vi "Watlow.vi"() -> ()   [LabVIEW 2017]
uses:
  dll/Watbus.dll
  Type Def/Data.ctl
panel:
  out "Cool bench":dbl caption="Cool" format="%#_5g"
  out "Heat bench":dbl caption="Heat" format="%#_5g"
  out "Cool tripleur":dbl caption="Cool" format="%#_5g"
  out "Heat tripleur":dbl caption="Heat" format="%#_5g"
  out "Cool doubleur":dbl caption="Cool" format="%#_5g"
  out "Heat doubleur":dbl caption="Heat" format="%#_5g"
  out "COM port":i64
  out "error?":bool caption="erreur ?"
  out "User file contents Watlow":dbl[](array[numeric])
  out "file path":path
  out "valeur de l'horloge en ms":u32
  in  "Bouton Accueil":bool
  out "sortie d'erreur":errorcluster
  out "IsConnected":bool
  out "ILabVIEW":refnum<k24>
  out "error out 2":errorcluster
  out "Chaîne":string
  out "error IO":errorcluster
  out "Communications Port":refnum<visa-resource-name>
  in  "Start":bool
  out "Watlow file (1sec)":refnum<file>
  out "Tableau":dbl[][](array[numeric])
  out "Bench":dbl format="%#_5g"
  out "THG":dbl format="%#_5g"
  out "SHG":dbl format="%#_5g"
  in  "Stop":bool
  out "error out":errorcluster caption="sortie d'erreur"
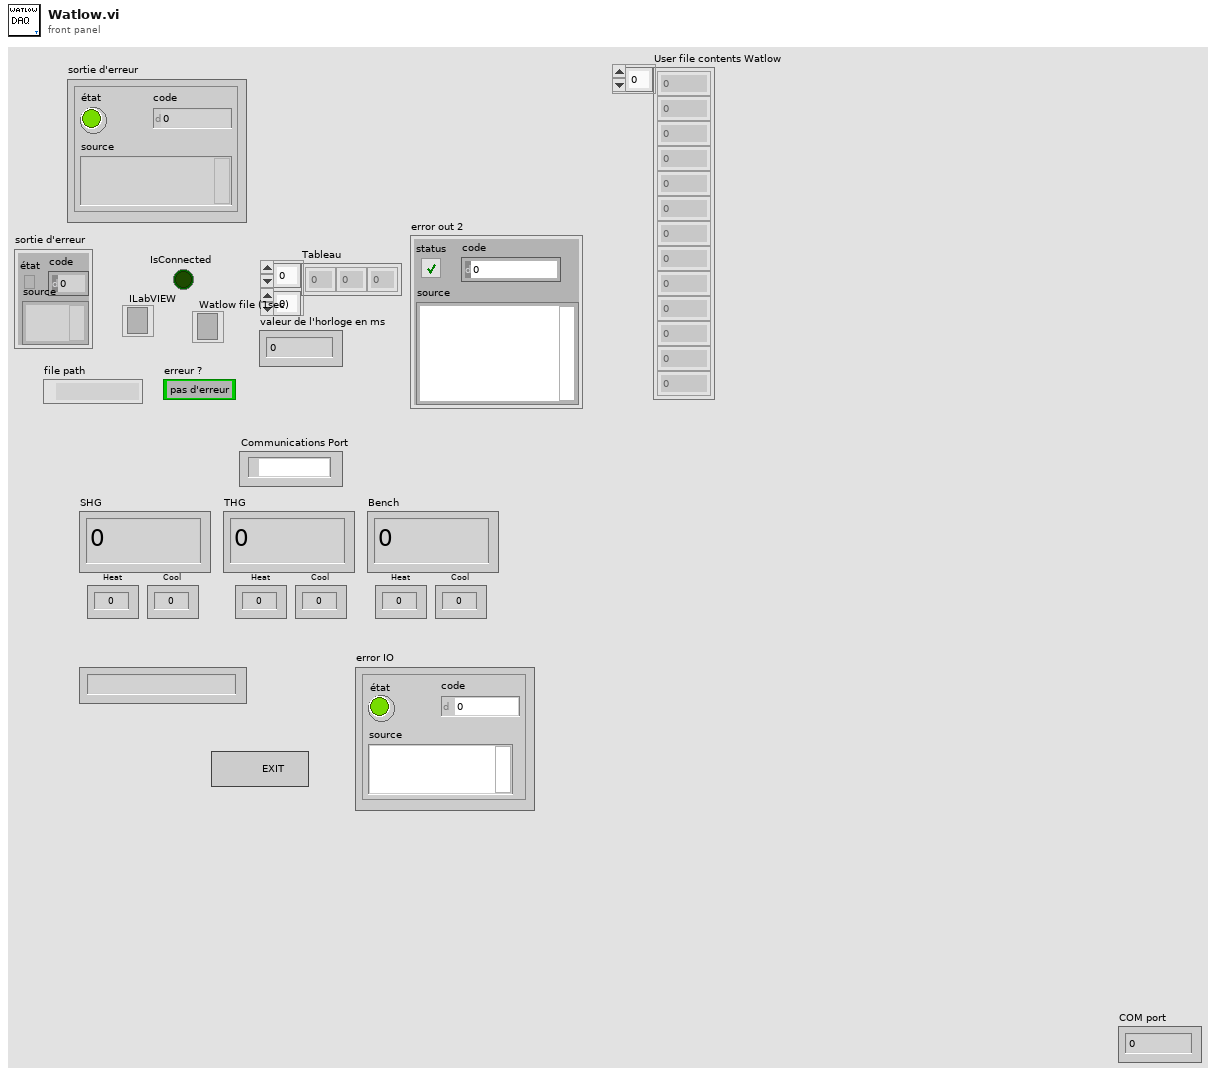
[diagram p1: front panel]
types:
  T1 = enum8{"Enabled", "Disabled", "Disabled and Grayed Out"}
  T2 = typedef "Data.ctl" = cluster{"Enum":enum16{"Init", "Read", "Stop"}, "Tableau":dbl[], "Date":string, "Time":u32}
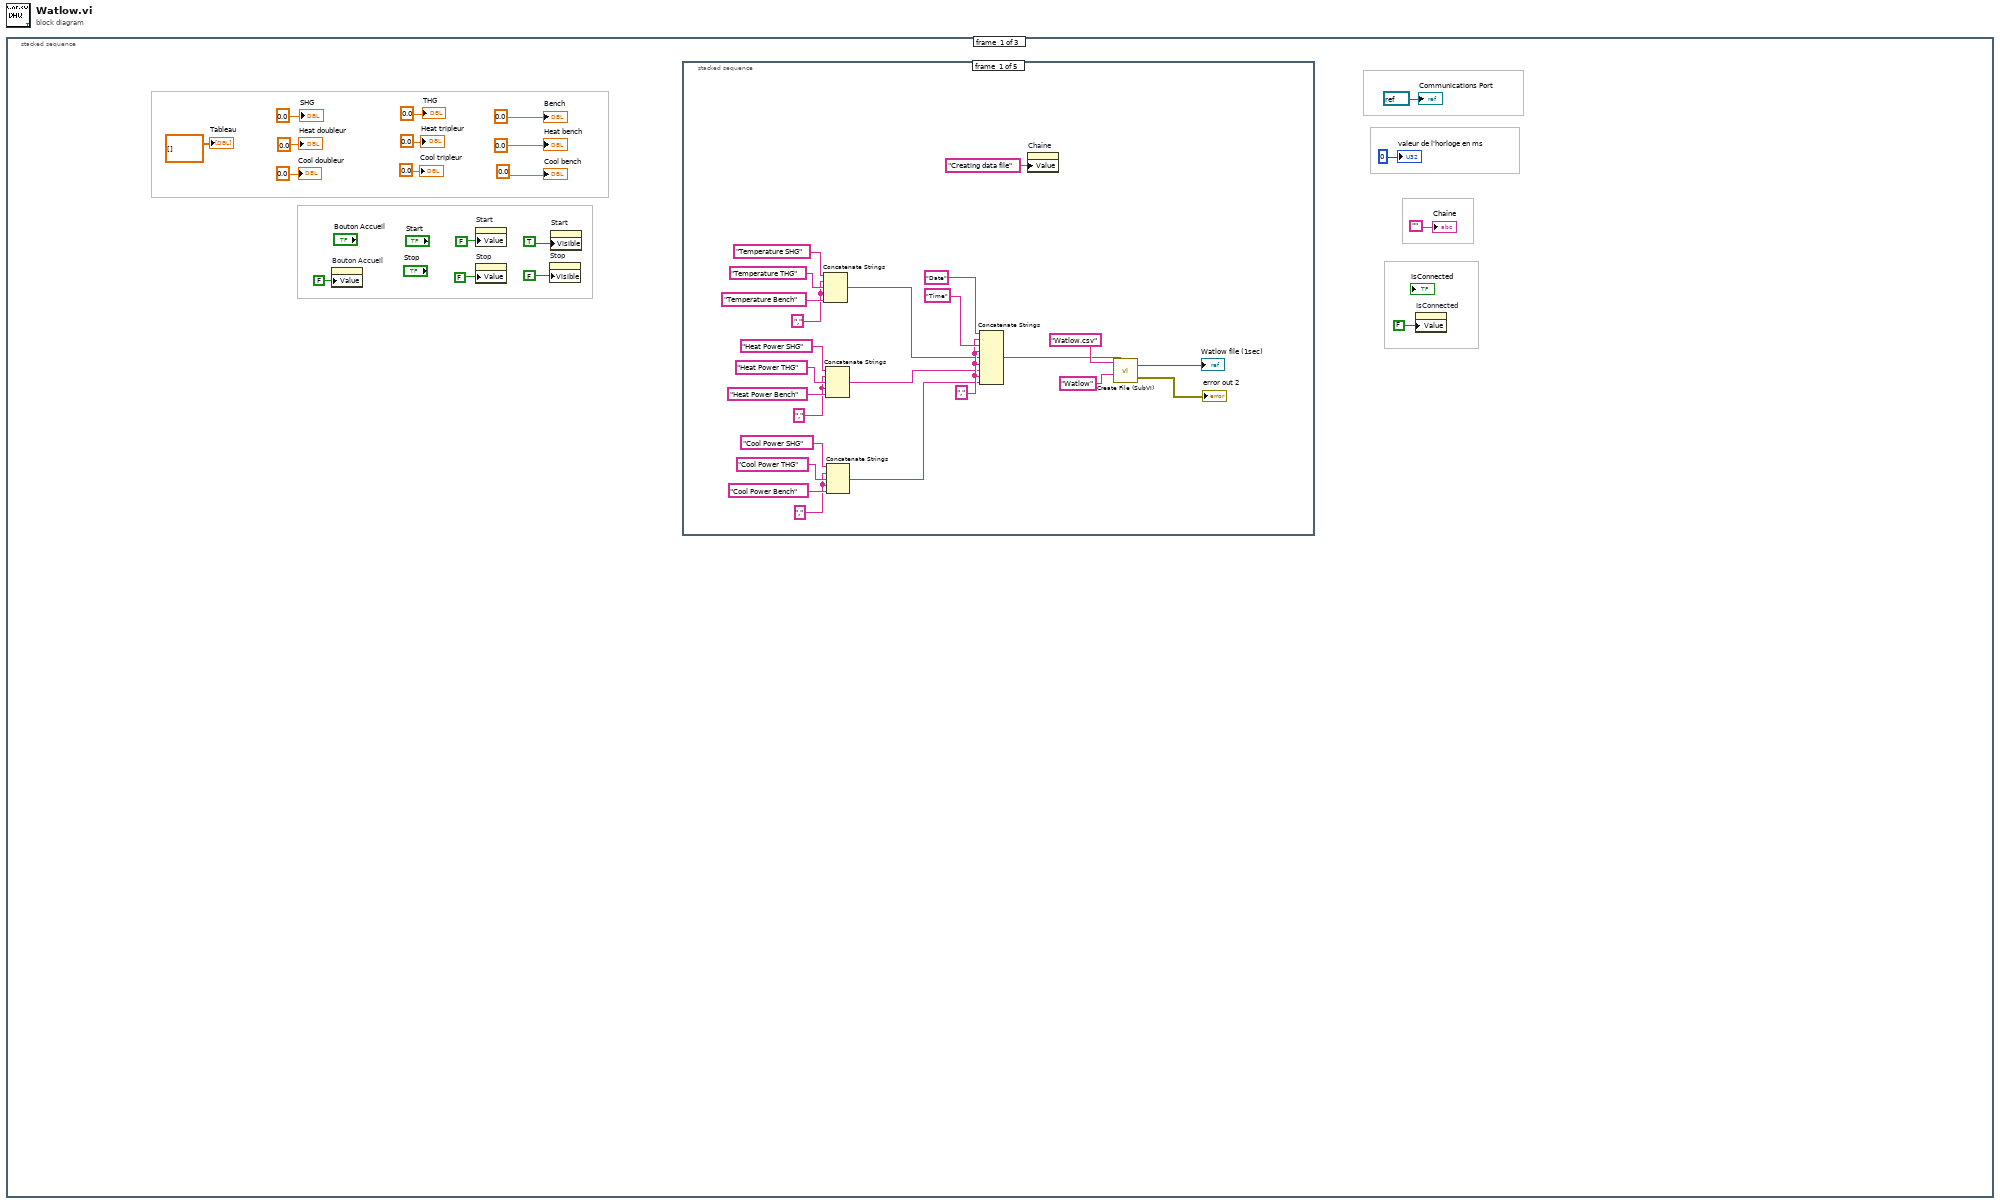
[diagram p0: block diagram]
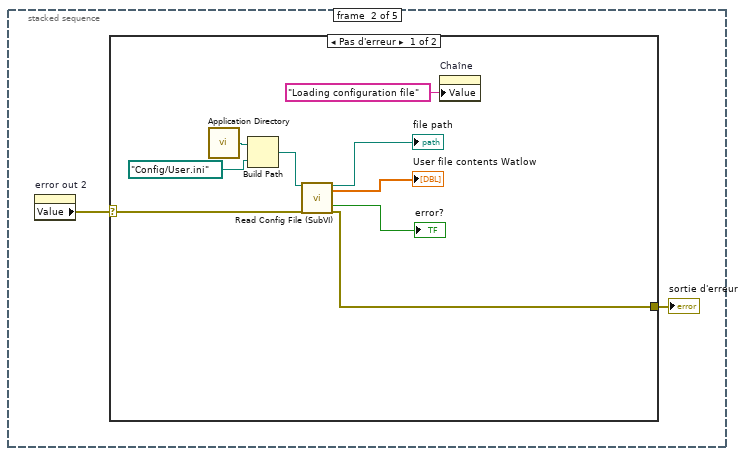
[diagram p2: hidden frame]
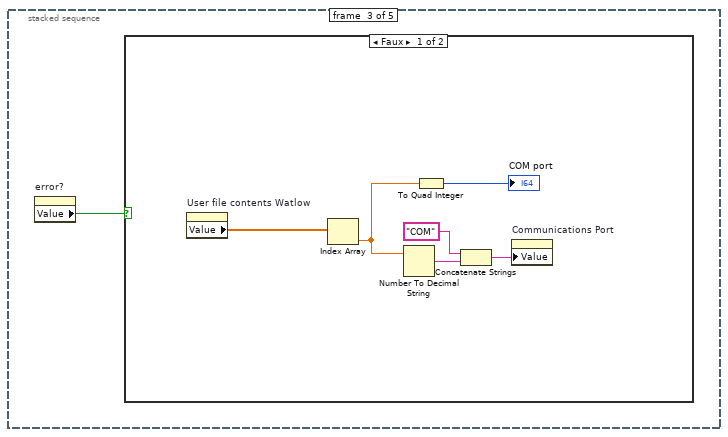
[diagram p4: hidden frame]
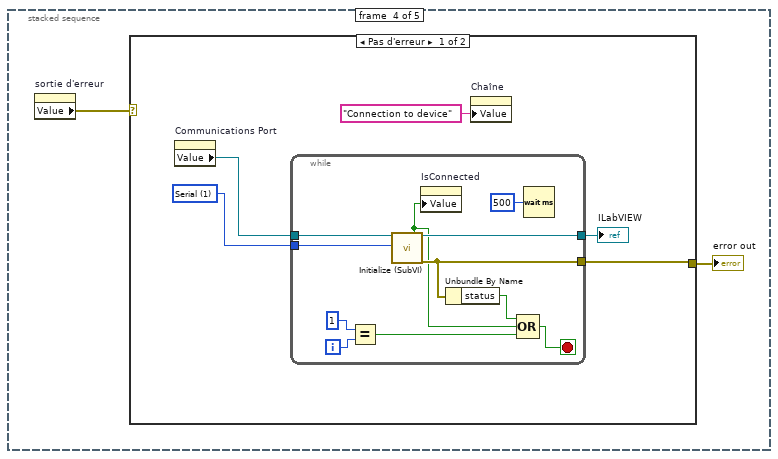
[diagram p6: hidden frame]
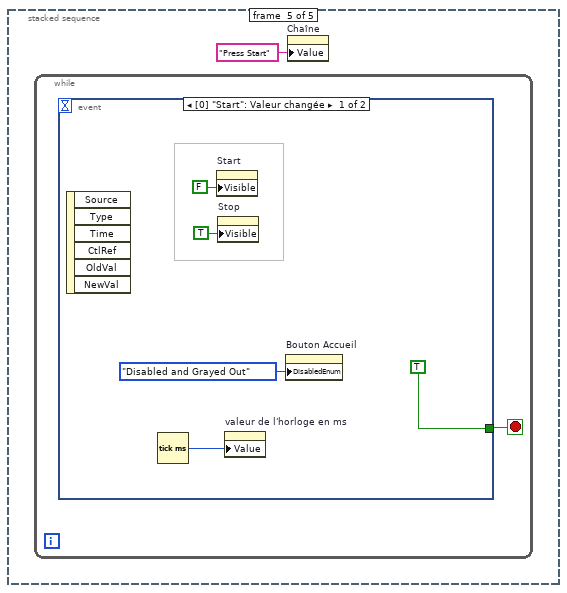
[diagram p8: hidden frame]
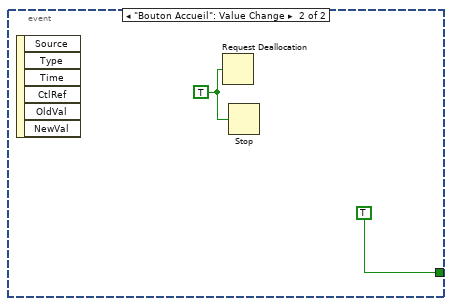
[diagram p9: hidden frame]
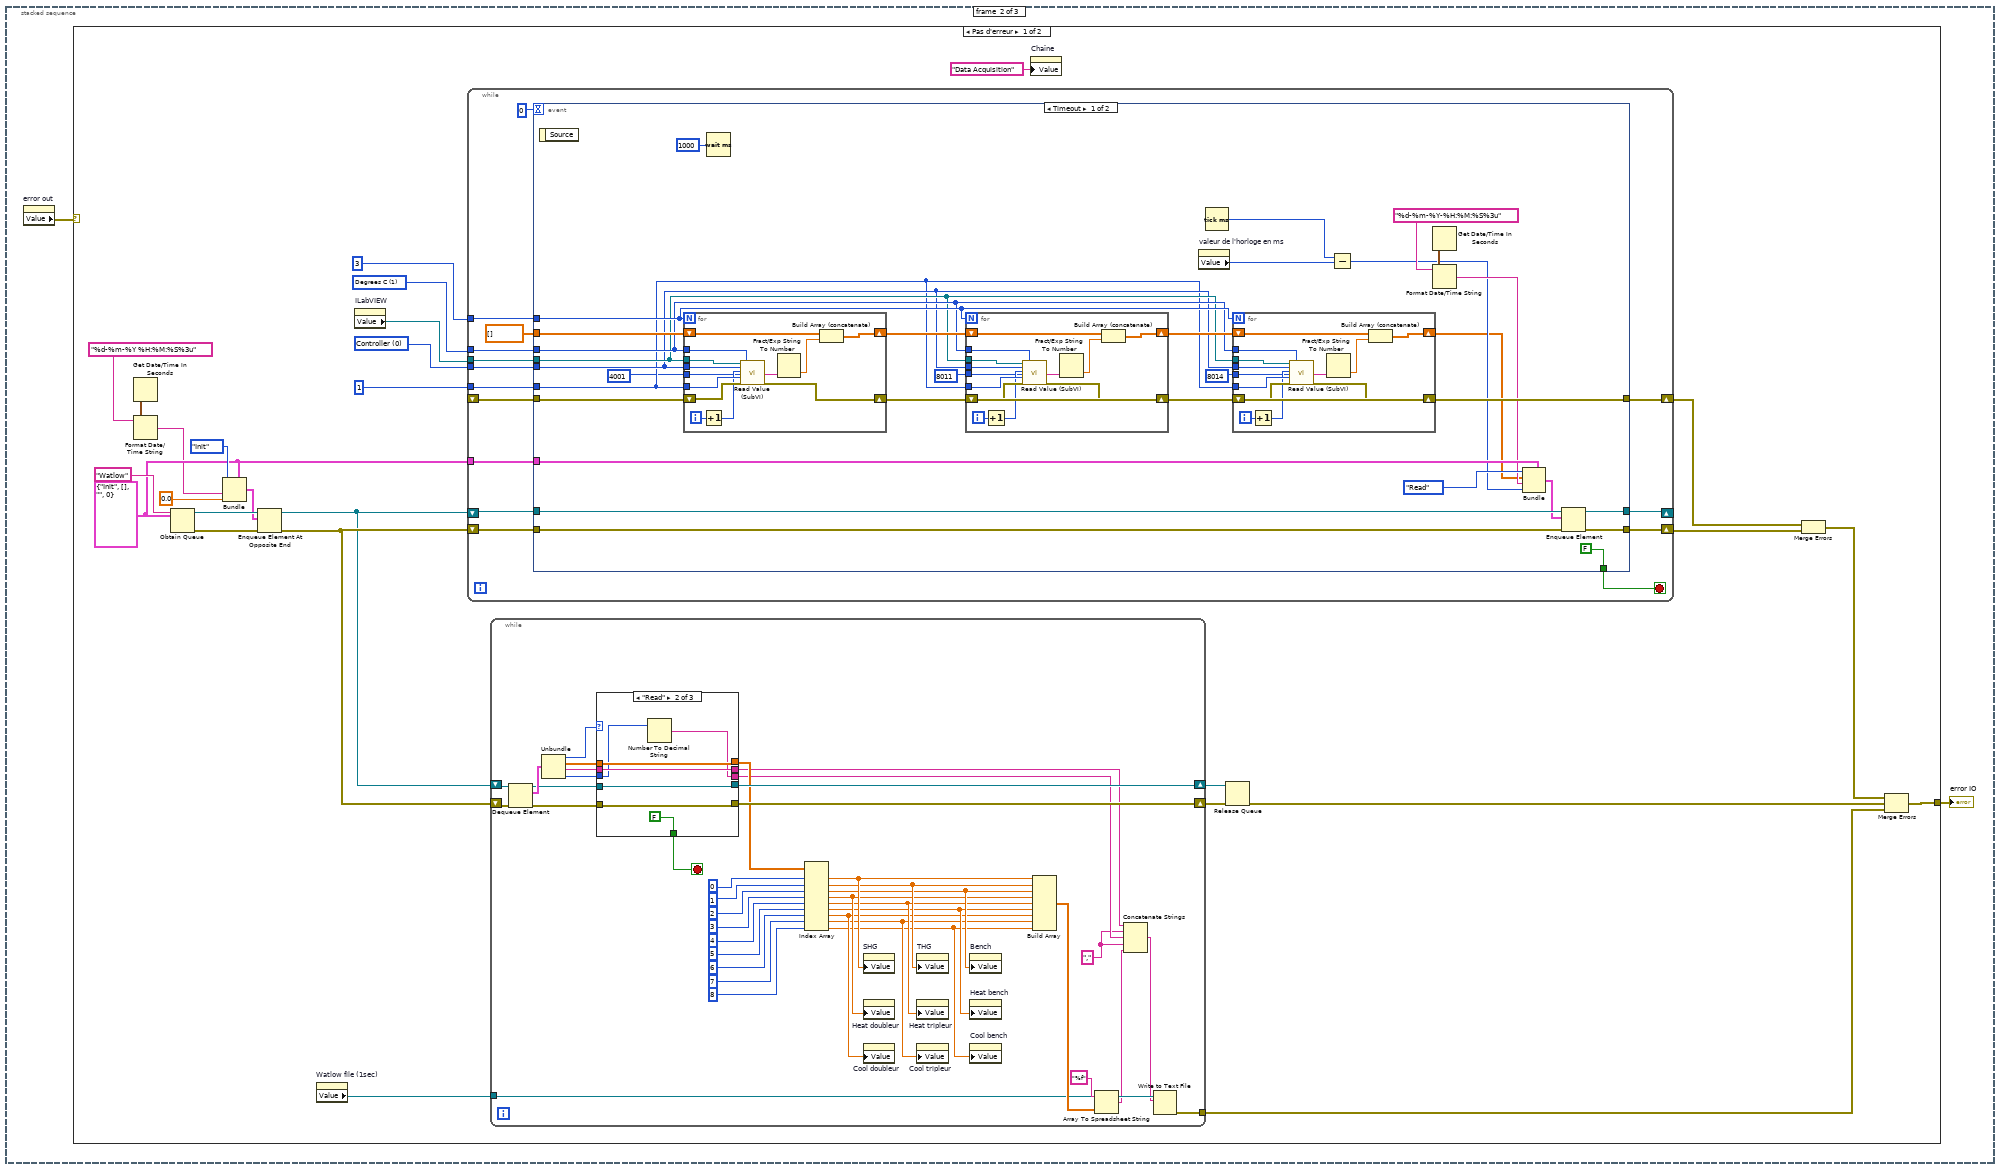
[diagram p10: hidden frame]
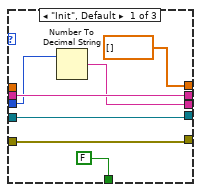
[diagram p11: hidden frame]
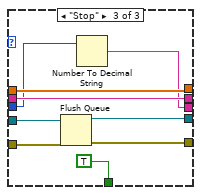
[diagram p12: hidden frame]
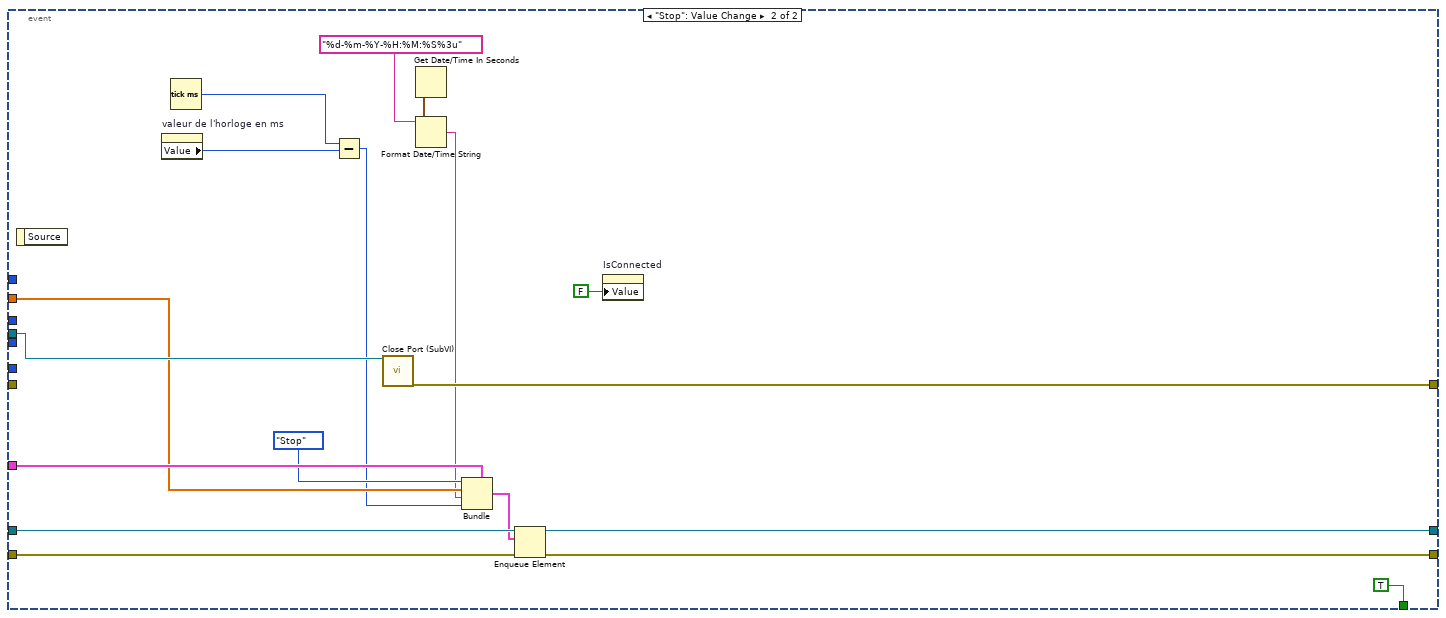
[diagram p13: hidden frame]
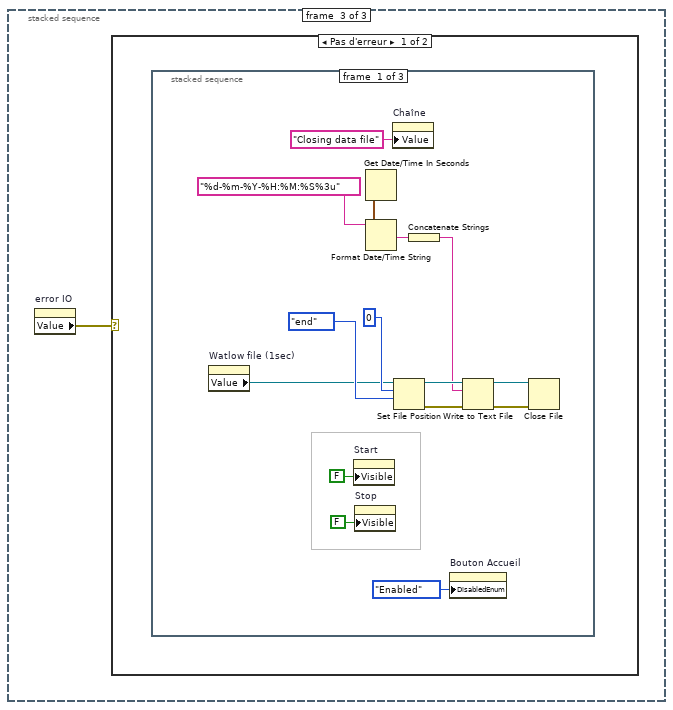
[diagram p15: hidden frame]
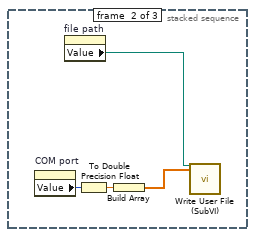
[diagram p16: hidden frame]
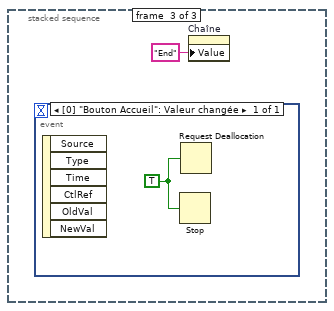
[diagram p17: hidden frame]
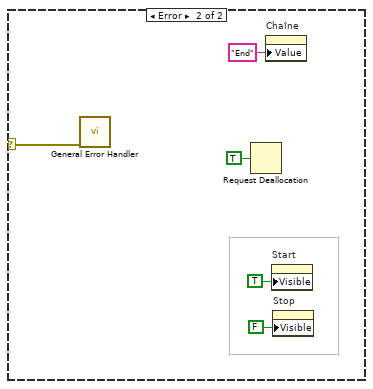
[diagram p18: hidden frame]
diagram:
  n1 = stacked-sequence {
    frame #0 {
      n2 = property on="Bouton Accueil" class="Bool (strict)"("Value"=FALSE ("Bouton Accueil")) -> ()  [unwired: 2 in, 2 out]
      n3 = property on="Start" class="Bool (strict)"("Value"=FALSE ("Start")) -> ()  [unwired: 2 in, 2 out]
      n4 = property on="Stop" class="Bool (strict)"("Value"=FALSE ("Bouton Stop")) -> ()  [unwired: 2 in, 2 out]
      n5 = property on="Stop" class="Bool (strict)"("Visible"=FALSE) -> ()  [unwired: 2 in, 2 out]
      n6 = property on="Start" class="Bool (strict)"("Visible"=TRUE) -> ()  [unwired: 2 in, 2 out]
      n7 = stacked-sequence {
        frame #0 {
          w22 = ","
          w26 = ","
          w31 = ","
          w36 = ","
          n8 = Concatenate Strings("Temperature SHG" ("chaîne"), w31, "Temperature THG" ("chaîne"), w31, "Temperature Bench" ("chaîne")) -> (w30:string)
          n9 = Concatenate Strings("Heat Power SHG" ("chaîne"), w26, "Heat Power THG" ("chaîne"), w26, "Heat Power Bench" ("chaîne")) -> (w21:string)
          n10 = Concatenate Strings("Cool Power SHG" ("chaîne"), w22, "Cool Power THG" ("chaîne"), w22, "Cool Power Bench" ("chaîne")) -> (w20:string)
          n11 = Concatenate Strings("Date" ("chaîne"), w36, "Time" ("chaîne"), w36, w30, w36, w21, w36, w20) -> (w38:string)
          n12 = property on="Chaîne" class="Ch"("Value"="Creating data file" ("Chaîne")) -> ()  [unwired: 2 in, 2 out]
          n13 = call "Create File (SubVI).vi"("headers"="Watlow" ("data name"), "data name"=w38, "file name"="Watlow.csv") -> ("error out"=→"error out 2":errorcluster, "Byte Stream File out"=→"Watlow file (1sec)":refnum<file>)  [unwired: 1 in]
        }
        frame #1 {
          n14 = property on="error out 2" class="Clust (strict)"() -> ("Value"=w45:errorcluster)  [unwired: 2 in, 2 out]
          n15 = case shown="Pas d'erreur" w45 {
            selector: w45 -> [w53 w55]
            tunnel: [w47 w55] -> w44
            frame No Error {
              n16 = call <vilib>:"Application Directory.vi"() -> ("Application Directory"=w52:path)
              n17 = Build Path(base path=w52, name or relative path=path "Config/User.ini") -> (appended path=w50:path)
              n18 = call "Read Config File (SubVI).vi"("configuration file path"=w50, "entrée d'erreur (pas d'erreur)"=w53) -> ("file path"=→"file path":path, "User file contents Watlow"=→"User file contents Watlow":dbl[], "error?"=→"error?":bool, "sortie d'erreur"=w47:errorcluster)  [unwired: 14 in]
              n19 = property on="Chaîne" class="Ch"("Value"="Loading configuration file" ("Chaîne")) -> ()  [unwired: 2 in, 2 out]
            }
            frame Error {
            }
          }
          "sortie d'erreur" <- w44
        }
        frame #2 {
          n20 = property on="error?" class="Bool (strict)"() -> ("Value"=w56:bool)  [unwired: 2 in, 2 out]
          n21 = case shown="Faux" w56 {
            frame False {
              n22 = property on="User file contents Watlow" class="Tabl (strict)"() -> ("Value"=w62:dbl[])  [unwired: 2 in, 2 out]
              n23 = Index Array(array=w62) -> (element=w58:dbl)  [unwired: 1 in]
              n24 = Number To Decimal String(number=w58) -> (decimal integer string=w60:string)  [unwired: 1 in]
              n25 = To Quad Integer(1:w58) -> (0:→"COM port":i64)
              n26 = Concatenate Strings("COM" ("string"), w60) -> (w57:string)
              n27 = property on="Communications Port" class="NomVISA"("Value"=w57) -> ()  [unwired: 2 in, 2 out]
            }
            frame True {
            }
          }
        }
        frame #3 {
          n28 = property on="sortie d'erreur" class="Clust (strict)"() -> ("Value"=w63:errorcluster)  [unwired: 2 in, 2 out]
          n29 = case shown="Pas d'erreur" w63 {
            selector: w63 -> [_ w81]
            tunnel: [w67 w81] -> w64
            frame No Error {
              w69 = 1 items=["Usb", "Serial", "Ethernet", "Unconnected"] ("InterfaceType")
              n30 = property on="Communications Port" class="NomVISA"() -> ("Value"=w65:refnum<visa-resource-name>)  [unwired: 2 in, 2 out]
              n31 = while {
                tunnel: [w73] -> w67
                tunnel: w69 -> [w80]
                tunnel: w65 -> [w71]
                tunnel: [w74] -> w66
                i -> [w78]
                stop <- w79 stop-if-true
                n32 = Equal?(x=1, y=w78) -> (x = y?=w76:bool)
                n33 = call "Initialize (SubVI).vi"("Communications Port"=w71, "InterfaceType"=w80) -> ("IsConnected"=w70:bool, "ILabVIEW"=w74:refnum<k24>, "error out"=w73:errorcluster)  [unwired: 15 in]
                n34 = property on="IsConnected" class="Bool (strict)"("Value"=w70) -> ()  [unwired: 2 in, 2 out]
                n35 = Unbundle By Name(w73) -> ("status"=w72:bool)
                n36 = Compound Arithmetic op=OR ("Opérateur arithmétique")(w72, w70, w76) -> (w79:bool)
                n37 = Wait (ms)(milliseconds to wait=u32 500 ("attente (ms)")) -> ()  [unwired: 1 out]
              }
              "ILabVIEW" <- w66
              n38 = property on="Chaîne" class="Ch"("Value"="Connection to device" ("Chaîne")) -> ()  [unwired: 2 in, 2 out]
            }
            frame Error {
            }
          }
          "error out" <- w64
        }
        frame #4 {
          n39 = while {
            stop <- w83 stop-if-true
            n40 = event shown="[0] \"Start\": Valeur changée" {
              selector: _ -> [_ _]
              dyn-events: _ -> [_ _]
              timeout: _ -> [_ _]
              tunnel: [TRUE TRUE] -> w83
              event "Start": Value Change {
                n41 = event-data() -> ()  [unwired: 1 in, 6 out]
                n42 = Tick Count (ms)() -> (millisecond timer value=w84:u32)
                n43 = property on="Start" class="Bool (strict)"("Visible"=FALSE) -> ()  [unwired: 2 in, 2 out]
                n44 = property on="Stop" class="Bool (strict)"("Visible"=TRUE) -> ()  [unwired: 2 in, 2 out]
                n45 = property on="valeur de l'horloge en ms" class="NumNb (strict)"("Value"=w84) -> ()  [unwired: 2 in, 2 out]
                n46 = property on="Bouton Accueil" class="Bool (strict)"("DisabledEnum"=T1."Disabled and Grayed Out" ("Désactivé")) -> ()  [unwired: 2 in, 2 out]
              }
              event "Bouton Accueil": Value Change {
                w90 = TRUE ("flag")
                n47 = event-data() -> ()  [unwired: 1 in, 6 out]
                n48 = Request Deallocation(w90) -> ()
                n49 = Stop(stop? (T)=w90) -> ()
              }
            }
          }
          n50 = property on="Chaîne" class="Ch"("Value"="Press Start" ("Chaîne")) -> ()  [unwired: 2 in, 2 out]
        }
      }
      n51 = property on="IsConnected" class="Bool (strict)"("Value"=FALSE ("IsConnected")) -> ()  [unwired: 2 in, 2 out]
      "SHG" <- 0.0 ("élément")
      "THG" <- 0.0 ("élément 2")
      "Bench" <- 0.0 ("élément 3")
      "Tableau" <- dbl[][] [] ("Tableau")
      "Chaîne" <- ""
      "Communications Port" <- refnum<visa-resource-name> refnum ("Communications Port")
      "valeur de l'horloge en ms" <- u32 0 ("valeur de l'horloge en ms")
      "Heat doubleur" <- 0.0 ("Heat doubleur")
      "Cool doubleur" <- 0.0 ("Cool doubleur")
      "Heat tripleur" <- 0.0 ("Heat tripleur")
      "Cool tripleur" <- 0.0 ("Cool tripleur")
      "Heat bench" <- 0.0 ("Heat bench")
      "Cool bench" <- 0.0 ("Cool bench")
    }
    frame #1 {
      n52 = property on="error out" class="Clust (strict)"() -> ("Value"=w92:errorcluster)  [unwired: 2 in, 2 out]
      n53 = case shown="Pas d'erreur" w92 {
        selector: w92 -> [_ w284]
        tunnel: [w106 w284] -> w91
        frame No Error {
          w117 = 0 items=["Controller", "RUI", "PC", "CommsCard"] ("DeviceType")
          w118 = u8 1 items=["Degrees F", "Degrees C"] ("TemperatureUnits")
          w97 = T2 {"Enum"=enum."Init", "Tableau"=[], "Date"="", "Time"=0} ("Enum")
          n54 = Get Date/Time In Seconds() -> (seconds since 1Jan1904=w96:timestamp)
          n55 = Format Date/Time String(time format string (%c)="%d-%m-%Y %H:%M:%S%3u", seconds (now)=w96) -> (date/time string=w94:string)  [unwired: 1 in]
          n56 = Obtain Queue(name (unnamed)="Watlow" ("nom (aucun)"), element data type=w97) -> (queue out=w100:refnum<queue>, error out=w103:errorcluster)  [unwired: 3 in, 1 out]
          n57 = Bundle(cluster=w97, "Enum"=enum16{"Init", "Read", "Stop"}."Init", "Date"=w94, "Time"=0.0) -> (w98:T2)  [unwired: 1 in]
          n58 = Enqueue Element At Opposite End(queue=w100, element=w98, error in (no error)=w103) -> (queue out=w101:refnum<queue>, error out=w102:errorcluster)  [unwired: 1 in, 1 out]
          n59 = property on="Watlow file (1sec)" class="Ref (strict)"() -> ("Value"=w107:refnum<file>)  [unwired: 2 in, 2 out]
          n60 = property on="ILabVIEW" class="Ref (strict)"() -> ("Value"=w104:refnum<k24>)  [unwired: 2 in, 2 out]
          n61 = while {
            shift-right: [w196] -> w111
            shift-left: w102 -> [w197]
            shift-right: [w194] -> _
            shift-left: w101 -> [w195]
            tunnel: w118 -> [w193]
            tunnel: w117 -> [w192]
            tunnel: 1 ("InstanceId") -> [w191]
            tunnel: 3 -> [w190]
            shift-right: [w188] -> w112
            shift-left: _ -> [w189]
            tunnel: w97 -> [w187]
            tunnel: w104 -> [w184]
            stop <- w186 stop-if-true
            n62 = event shown="[0] Timeout" {
              selector: _ -> [_ _]
              dyn-events: _ -> [_ _]
              timeout: 0 -> [_ _]
              tunnel: w197 -> [w224 w281]
              tunnel: [w223 w280] -> w196
              tunnel: w195 -> [w226 w282]
              tunnel: [w225 w279] -> w194
              tunnel: w193 -> [w204 _]
              tunnel: w192 -> [w202 _]
              tunnel: w191 -> [w201 _]
              tunnel: w190 -> [w208 _]
              tunnel: w189 -> [w222 _]
              tunnel: [w221 w275] -> w188
              tunnel: w187 -> [w220 w277]
              tunnel: [FALSE TRUE] -> w186
              tunnel: w184 -> [w203 w274]
              tunnel: dbl[] [] -> [w216 w272]
              event Timeout {
                n63 = event-data() -> ()  [unwired: 1 in, 1 out]
                n64 = for {
                  N: w208 -> [_]
                  tunnel: w204 -> [w265]
                  tunnel: w202 -> [w264]
                  tunnel: w201 -> [w263]
                  shift-right: [w260] -> w221
                  shift-left: w222 -> [w261]
                  shift-right: [w256] -> w205
                  shift-left: w216 -> [w255]
                  tunnel: w203 -> [w254]
                  tunnel: 4001 ("ParameterID") -> [w253]
                  i -> [w262]
                  n65 = Increment(x=w262) -> (x+1=w258:i32)
                  n66 = call "Read Value (SubVI).vi"("ILabVIEW In"=w254, "DeviceType"=w264, "Zone"=w258, "ParameterID"=w253, "InstanceId"=w263, "error in (no error)"=w261, "TemperatureUnits"=w265) -> ("Value Out"=w259:string, "error out"=w260:errorcluster)  [unwired: 10 in, 1 out]
                  n67 = Fract/Exp String To Number(string=w259) -> (number=w257:dbl)  [unwired: 3 in, 1 out]
                  n68 = Build Array (concatenate)(w255, w257) -> (w256:dbl[])
                }
                n69 = Wait (ms)(milliseconds to wait=u32 1000 ("attente (ms)")) -> ()  [unwired: 1 out]
                n70 = for {
                  N: w208 -> [_]
                  tunnel: w204 -> [w252]
                  tunnel: w202 -> [w251]
                  tunnel: w201 -> [w250]
                  shift-right: [w247] -> _
                  shift-left: _ -> [w248]
                  shift-right: [w243] -> w206
                  shift-left: w205 -> [w242]
                  tunnel: w203 -> [w241]
                  tunnel: 8011 -> [w240]
                  i -> [w249]
                  n71 = Increment(x=w249) -> (x+1=w245:i32)
                  n72 = call "Read Value (SubVI).vi"("ILabVIEW In"=w241, "DeviceType"=w251, "Zone"=w245, "ParameterID"=w240, "InstanceId"=w250, "error in (no error)"=w248, "TemperatureUnits"=w252) -> ("Value Out"=w246:string, "error out"=w247:errorcluster)  [unwired: 10 in, 1 out]
                  n73 = Fract/Exp String To Number(string=w246) -> (number=w244:dbl)  [unwired: 3 in, 1 out]
                  n74 = Build Array (concatenate)(w242, w244) -> (w243:dbl[])
                }
                n75 = property on="valeur de l'horloge en ms" class="NumNb (strict)"() -> ("Value"=w211:u32)  [unwired: 2 in, 2 out]
                n76 = Tick Count (ms)() -> (millisecond timer value=w212:u32)
                n77 = for {
                  N: w208 -> [_]
                  tunnel: w204 -> [w239]
                  tunnel: w202 -> [w238]
                  tunnel: w201 -> [w237]
                  shift-right: [w234] -> _
                  shift-left: _ -> [w235]
                  shift-right: [w230] -> w207
                  shift-left: w206 -> [w229]
                  tunnel: w203 -> [w228]
                  tunnel: 8014 -> [w227]
                  i -> [w236]
                  n78 = Increment(x=w236) -> (x+1=w232:i32)
                  n79 = call "Read Value (SubVI).vi"("ILabVIEW In"=w228, "DeviceType"=w238, "Zone"=w232, "ParameterID"=w227, "InstanceId"=w237, "error in (no error)"=w235, "TemperatureUnits"=w239) -> ("Value Out"=w233:string, "error out"=w234:errorcluster)  [unwired: 10 in, 1 out]
                  n80 = Fract/Exp String To Number(string=w233) -> (number=w231:dbl)  [unwired: 3 in, 1 out]
                  n81 = Build Array (concatenate)(w229, w231) -> (w230:dbl[])
                }
                n82 = Subtract(x=w212, y=w211) -> (x-y=w210:u32)
                n83 = Get Date/Time In Seconds() -> (seconds since 1Jan1904=w215:timestamp)
                n84 = Format Date/Time String(time format string (%c)="%d-%m-%Y-%H:%M:%S%3u", seconds (now)=w215) -> (date/time string=w213:string)  [unwired: 1 in]
                n85 = Bundle(cluster=w220, "Enum"=enum16{"Init", "Read", "Stop"}."Read", "Tableau"=w207, "Date"=w213, "Time"=w210) -> (w219:T2)
                n86 = Enqueue Element(queue=w226, element=w219, error in (no error)=w224) -> (queue out=w225:refnum<queue>, error out=w223:errorcluster)  [unwired: 1 in, 1 out]
              }
              event "Stop": Value Change {
                n87 = event-data() -> ()  [unwired: 1 in, 1 out]
                n88 = property on="valeur de l'horloge en ms" class="NumNb (strict)"() -> ("Value"=w267:u32)  [unwired: 2 in, 2 out]
                n89 = Tick Count (ms)() -> (millisecond timer value=w268:u32)
                n90 = Subtract(x=w268, y=w267) -> (x-y=w266:u32)
                n91 = call "Close Port (SubVI).vi"("ILabVIEW In"=w274) -> ("error out"=w275:errorcluster)  [unwired: 18 in]
                n92 = Get Date/Time In Seconds() -> (seconds since 1Jan1904=w271:timestamp)
                n93 = Format Date/Time String(time format string (%c)="%d-%m-%Y-%H:%M:%S%3u", seconds (now)=w271) -> (date/time string=w269:string)  [unwired: 1 in]
                n94 = Bundle(cluster=w277, "Enum"=enum16{"Init", "Read", "Stop"}."Stop", "Tableau"=w272, "Date"=w269, "Time"=w266) -> (w278:T2)
                n95 = Enqueue Element(queue=w282, element=w278, error in (no error)=w281) -> (queue out=w279:refnum<queue>, error out=w280:errorcluster)  [unwired: 1 in, 1 out]
                n96 = property on="IsConnected" class="Bool (strict)"("Value"=FALSE ("IsConnected")) -> ()  [unwired: 2 in, 2 out]
              }
            }
          }
          n97 = while {
            shift-right: [w151] -> w114
            shift-left: w101 -> [w158]
            shift-right: [w152] -> w113
            shift-left: w102 -> [w159]
            tunnel: [w143] -> w108
            tunnel: w107 -> [w142]
            stop <- w150 stop-if-true
            w135 = ","
            n98 = Dequeue Element(queue=w158, error in (no error)=w159) -> (queue out=w154:refnum<queue>, element=w157:T2, error out=w153:errorcluster)  [unwired: 1 in, 1 out]
            n99 = Unbundle(w157) -> ("Enum"=w156:enum16{"Init", "Read", "Stop"}, "Tableau"=w155:dbl[], "Date"=w140:string, "Time"=w139:u32)
            n100 = case shown="\"Read\"" w156 {
              tunnel: w155 -> [_ w170 w177]
              tunnel: w154 -> [w166 w173 w182]
              tunnel: w153 -> [w165 w172 w181]
              tunnel: [w165 w172 w180] -> w152
              tunnel: [w166 w173 w179] -> w151
              tunnel: [FALSE FALSE TRUE] -> w150
              tunnel: [dbl[] [] w170 w177] -> w146
              tunnel: [w162 w169 w176] -> w137
              tunnel: w140 -> [w162 w169 w176]
              tunnel: w139 -> [w161 w168 w175]
              tunnel: [w160 w167 w174] -> w138
              frame "Init", Default {
                n101 = Number To Decimal String(number=w161) -> (decimal integer string=w160:string)  [unwired: 1 in]
              }
              frame "Read" {
                n102 = Number To Decimal String(number=w168) -> (decimal integer string=w167:string)  [unwired: 1 in]
              }
              frame "Stop" {
                n103 = Flush Queue(queue=w182, error in (no error)=w181) -> (queue out=w179:refnum<queue>, error out=w180:errorcluster)  [unwired: 1 out]
                n104 = Number To Decimal String(number=w175) -> (decimal integer string=w174:string)  [unwired: 1 in]
              }
            }
            n105 = Index Array(array=w146, index #1=0 ("indice"), index #2=1 ("indice"), index #3=2 ("indice"), index #4=3 ("indice"), index #5=4 ("indice"), index #6=5 ("indice"), index #7=6 ("indice"), index #8=7 ("indice"), index #9=8 ("indice")) -> (element #1=w128:dbl, element #2=w127:dbl, element #3=w126:dbl, element #4=w125:dbl, element #5=w124:dbl, element #6=w123:dbl, element #7=w122:dbl, element #8=w121:dbl, element #9=w120:dbl)
            n106 = property on="SHG" class="NumNb (strict)"("Value"=w128) -> ()  [unwired: 2 in, 2 out]
            n107 = property on="Heat doubleur" class="NumNb (strict)"("Value"=w125) -> ()  [unwired: 2 in, 2 out]
            n108 = property on="Cool doubleur" class="NumNb (strict)"("Value"=w122) -> ()  [unwired: 2 in, 2 out]
            n109 = property on="THG" class="NumNb (strict)"("Value"=w127) -> ()  [unwired: 2 in, 2 out]
            n110 = property on="Heat tripleur" class="NumNb (strict)"("Value"=w124) -> ()  [unwired: 2 in, 2 out]
            n111 = property on="Cool tripleur" class="NumNb (strict)"("Value"=w121) -> ()  [unwired: 2 in, 2 out]
            n112 = property on="Bench" class="NumNb (strict)"("Value"=w126) -> ()  [unwired: 2 in, 2 out]
            n113 = property on="Heat bench" class="NumNb (strict)"("Value"=w123) -> ()  [unwired: 2 in, 2 out]
            n114 = property on="Cool bench" class="NumNb (strict)"("Value"=w120) -> ()  [unwired: 2 in, 2 out]
            n115 = Build Array(w128, w127, w126, w125, w124, w123, w122, w121, w120) -> (w144:dbl[])
            n116 = Array To Spreadsheet String(array=w144, 3:"%f" ("chaîne de format")) -> (spreadsheet string=w136:string)  [unwired: 1 in]
            n117 = Concatenate Strings(w137, w135, w138, w135, w136) -> (w141:string)
            n118 = Write to Text File(file (use dialog)=w142, text=w141) -> (error out=w143:errorcluster)  [unwired: 2 in, 2 out]
          }
          n119 = property on="Chaîne" class="Ch"("Value"="Data Acquisition" ("Chaîne")) -> ()  [unwired: 2 in, 2 out]
          n120 = Release Queue(queue=w114, error in (no error)=w113) -> (error out=w110:errorcluster)  [unwired: 1 in, 2 out]
          n121 = Merge Errors(w112, w111) -> (w109:errorcluster)
          n122 = Merge Errors(w109, w110, w108) -> (w106:errorcluster)
        }
        frame Error {
        }
      }
      "error IO" <- w91
    }
    frame #2 {
      n123 = property on="error IO" class="Clust (strict)"() -> ("Value"=w285:errorcluster)  [unwired: 2 in, 2 out]
      n124 = case shown="Pas d'erreur" w285 {
        selector: w285 -> [_ w309]
        frame No Error {
          n125 = stacked-sequence {
            frame #0 {
              n126 = property on="Watlow file (1sec)" class="Ref (strict)"() -> ("Value"=w292:refnum<file>)  [unwired: 2 in, 2 out]
              n127 = property on="Start" class="Bool (strict)"("Visible"=FALSE) -> ()  [unwired: 2 in, 2 out]
              n128 = property on="Stop" class="Bool (strict)"("Visible"=FALSE) -> ()  [unwired: 2 in, 2 out]
              n129 = Get Date/Time In Seconds() -> (seconds since 1Jan1904=w298:timestamp)
              n130 = Format Date/Time String(time format string (%c)="%d-%m-%Y-%H:%M:%S%3u", seconds (now)=w298) -> (date/time string=w296:string)  [unwired: 1 in]
              n131 = property on="Chaîne" class="Ch"("Value"="Closing data file" ("Chaîne")) -> ()  [unwired: 2 in, 2 out]
              n132 = Set File Position(offset (in bytes) (0)=i64 0 ("offset (en octets) (0)"), refnum=w292, from (0:start)=enum16{"start", "end", "current"}."end" ("à partir de (0 : start)")) -> (refnum out=w299:refnum<file>, error out=w288:errorcluster)  [unwired: 1 in]
              n133 = Concatenate Strings(w296) -> (w295:string)
              n134 = property on="Bouton Accueil" class="Bool (strict)"("DisabledEnum"=T1."Enabled" ("Désactivé")) -> ()  [unwired: 2 in, 2 out]
              n135 = Write to Text File(file (use dialog)=w299, text=w295, error in=w288) -> (refnum out=w300:refnum<file>, error out=w287:errorcluster)  [unwired: 1 in, 1 out]
              n136 = Close File(refnum=w300, error in=w287) -> ()  [unwired: 2 out]
            }
            frame #1 {
              n137 = property on="COM port" class="NumNb (strict)"() -> ("Value"=w304:i64)  [unwired: 2 in, 2 out]
              n138 = property on="file path" class="Chm"() -> ("Value"=w301:path)  [unwired: 2 in, 2 out]
              n139 = To Double Precision Float(number=w304) -> (double precision float=w302:dbl)
              n140 = Build Array(w302) -> (w303:dbl[])
              n141 = call "Write User File (SubVI).vi"("configuration file path"=w301, "User file contents Watlow"=w303) -> ()  [unwired: 24 in, 2 out]
            }
            frame #2 {
              n142 = event shown="[0] \"Bouton Accueil\": Valeur changée" {
                selector: _ -> [_]
                dyn-events: _ -> [_]
                timeout: _ -> [_]
                event "Bouton Accueil": Value Change {
                  w306 = TRUE ("flag")
                  n143 = event-data() -> ()  [unwired: 1 in, 6 out]
                  n144 = Stop(stop? (T)=w306) -> ()
                  n145 = Request Deallocation(w306) -> ()
                }
              }
              n146 = property on="Chaîne" class="Ch"("Value"="End" ("Chaîne")) -> ()  [unwired: 2 in, 2 out]
            }
          }
        }
        frame Error {
          n147 = call <vilib>:"General Error Handler.vi"("error in (no error)"=w309) -> ()  [unwired: 10 in, 5 out]
          n148 = Request Deallocation(TRUE ("flag")) -> ()
          n149 = property on="Chaîne" class="Ch"("Value"="End" ("Chaîne")) -> ()  [unwired: 2 in, 2 out]
          n150 = property on="Start" class="Bool (strict)"("Visible"=TRUE) -> ()  [unwired: 2 in, 2 out]
          n151 = property on="Stop" class="Bool (strict)"("Visible"=FALSE) -> ()  [unwired: 2 in, 2 out]
        }
      }
    }
  }
